vi "CRYGet Interface Array.vi"(11 "N interfs":i32) -> (3 "Interface no Array":cluster{"String":string, "Value":ext}[](array[cluster]))   [LabVIEW 2013]
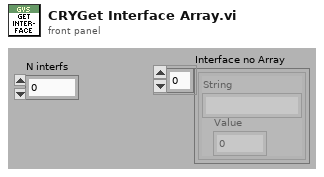
[diagram p1: front panel]
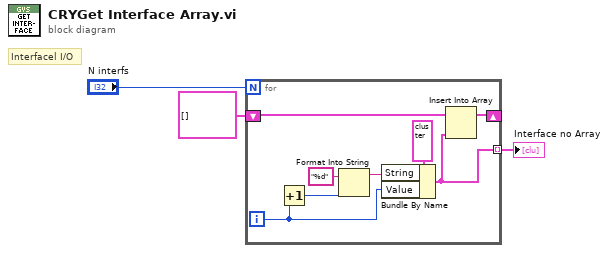
[diagram p0: block diagram]
diagram:
  # "Interfacel I/O"
  n1 = for {
    N: "N interfs" -> [_]
    shift-right: [w7] -> _
    shift-left: cluster{"String":string, "Value":ext}[] [] -> [w8]
    tunnel: [w4] -> w1 mode=indexing
    i -> [w6]
    n2 = Increment(x=w6) -> (x+1=w5:i32)
    n3 = Format Into String(format string="%d", w5) -> (resulting string=w10:string)  [unwired: 2 in, 1 out]
    n4 = Bundle By Name(cluster=cluster{"String":string, "Value":ext} {"String"="", "Value"=0.0}, "String"=w10, "Value"=w6) -> (w4:cluster{"String":string, "Value":ext})
    n5 = Insert Into Array(array=w8, new element=w4) -> (w7:cluster{"String":string, "Value":ext}[])  [unwired: 1 in]
  }
  "Interface no Array" <- w1
